vi "User Console.vi"(8 "error in (no error)":errorcluster, 10 "Queues":T3, 11 "UE Data Container":T4) -> (0 "error out":errorcluster)   [LabVIEW 2017]
doc: "The Process of ATM controller where user enters information and responds to system prompts.\n[Covers: UI1]"
uses:
  Shared Data/User Events/UE Data Container.ctl
  Error Handler/Controls/Error Data.ctl
  Controls/User Console - Transaction Enum.ctl
  Shared Data/Queues/Controls/Queues.ctl
  Controller/Controls/UI CMD.ctl
  Controller/Controls/Controller CMD.ctl
  Configuration/Controls/Config CMD.ctl
  Controls/User Console - Keypad.ctl
  Controls/User Console - Transactions.ctl
  Controls/User Console - References.ctl
panel:
  in  "Card Reader":bool
  in  "Transactions":T1
  in  "Keypad":T2
  # "[Covers: UI2]"
  # "[Covers: UI2B]"
  # "[Covers: UI2C]"
  # "[Covers: UI2A]"
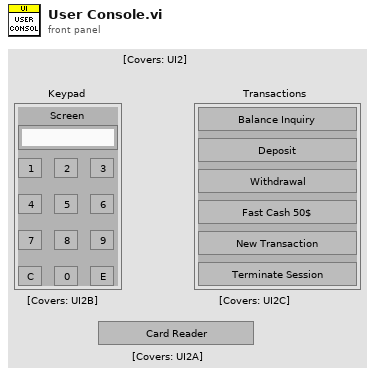
[diagram p1: front panel]
types:
  T1 = typedef "User Console - Transactions.ctl" = cluster{"Balance Inquiry":bool, "Deposit":bool, "Withdrawal":bool, "Fast Cash":bool, "New Transaction":bool, "Terminate":bool}
  T2 = typedef "User Console - Keypad.ctl" = cluster{"Screen":string, "1":bool, "2":bool, "3":bool, "4":bool, "5":bool, "6":bool, "7":bool, "8":bool, "9":bool, "C":bool, "0":bool, "E":bool}
  T3 = typedef "Queues.ctl" = cluster{"UI":refnum<queue>, "Controller":refnum<queue>, "Config":refnum<queue>, "User Console":refnum<queue>, "Display Console":refnum<queue>}
  T4 = typedef "UE Data Container.ctl" = cluster{"Stop UE":refnum<user-event>, "Stop DVR":refnum<data-value>, "Error UE":refnum<user-event>, "Deposit Change":refnum<user-event>, "Funds Change":refnum<user-event>, "Card Reader Change":refnum<user-event>, "Transaction Change":refnum<user-event>, "Keypad Screen Change":refnum<user-event>}
  T5 = typedef "User Console - References.ctl" = cluster{"Transactions":refnum<vi>, "Keypad":refnum<vi>, "Card Reader":refnum<vi>}
  T6 = typedef "User Console - Transaction Enum.ctl" = enum16{"Balance Inquiry", "Deposit", "Withdrawal", "Fat Cash", "New Transaction", "Terminate Session"}
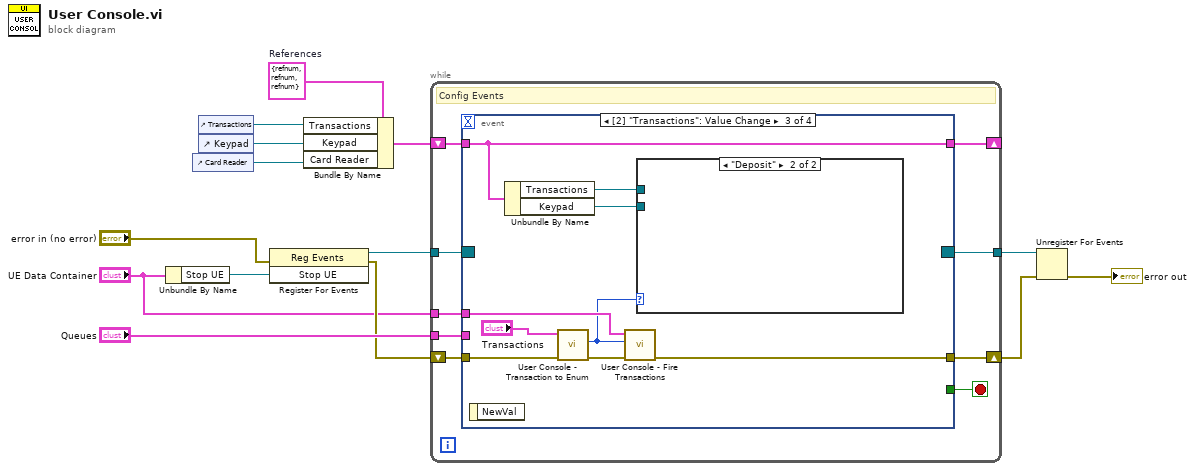
[diagram p0: block diagram]
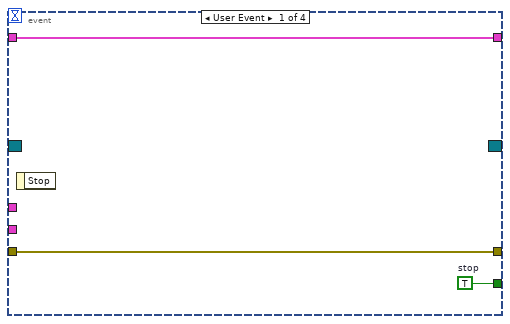
[diagram p2: hidden frame]
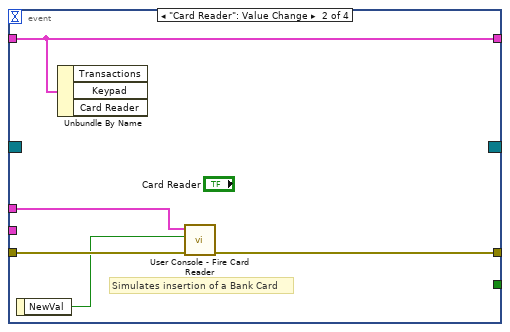
[diagram p3: hidden frame]
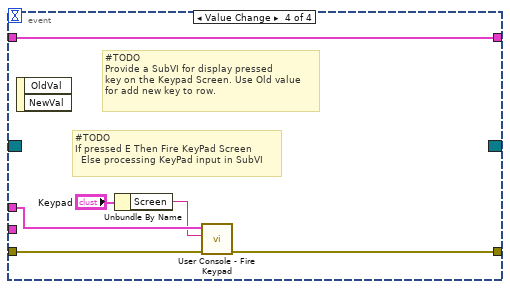
[diagram p5: hidden frame]
diagram:
  w6 = T5 {"Transactions"=refnum, "Keypad"=refnum, "Card Reader"=refnum}  # References
  n1 = Unbundle By Name("UE Data Container") -> ("Stop UE"=w14:refnum<user-event>)
  n2 = control-ref of="Card Reader"() -> (w3:refnum<vi>)
  n3 = control-ref of="Transactions"() -> (w5:refnum<vi>)
  n4 = control-ref of="Keypad"() -> (w4:refnum<vi>)
  n5 = register-events(error in="error in (no error)", w14) -> (reference out=w12:refnum<event-registration>, error out=w8:errorcluster)  [unwired: 1 in]
  n6 = Bundle By Name(cluster=w6, "Transactions"=w5, "Keypad"=w4, "Card Reader"=w3) -> (w2:T5)
  n7 = while {
    tunnel: w12 -> [w23]
    tunnel: [w22] -> w11
    tunnel: "Queues" -> [w20]
    shift-right: [w18] -> w10
    shift-left: w8 -> [w19]
    tunnel: "UE Data Container" -> [w17]
    shift-right: [w15] -> _
    shift-left: w2 -> [w16]
    stop <- w21 stop-if-true
    # "Config Events"
    n8 = event shown="[2] \"Transactions\": Value Change" {
      selector: w23 -> [_ _ _ _]
      dyn-events: [_ _ _ _] -> w22
      timeout: _ -> [_ _ _ _]
      tunnel: [w26 _ _ _] -> w21
      tunnel: w20 -> [_ _ _ _]
      tunnel: w19 -> [w24 w31 w40 w45]
      tunnel: [w24 w29 w37 w41] -> w18
      tunnel: w17 -> [_ w30 w39 w43]
      tunnel: w16 -> [w25 w27 w35 w46]
      tunnel: [w25 w27 w35 w46] -> w15
      event User Event {
        w26 = TRUE  # stop
        n9 = event-data() -> ()  [unwired: 1 in, 1 out]
      }
      event "Card Reader": Value Change {
        # "Simulates insertion of a Bank Card"
        n10 = event-data() -> ("NewVal"=w28:bool)  [unwired: 1 in]
        n11 = Unbundle By Name(w27) -> ()  [unwired: 3 out]
        n12 = call "User Console - Fire Card Reader.vi"("error in (no error)"=w31, "Card Reader Change"=w28, "UE Data Container"=w30) -> ("error out"=w29:errorcluster)  [unwired: 8 in]
      }
      event Value Change {
        n13 = event-data() -> ()  [unwired: 1 in, 1 out]
        n14 = Unbundle By Name(w35) -> ("Transactions"=w33:refnum<vi>, "Keypad"=w32:refnum<vi>)
        n15 = call "User Console - Transaction to Enum.vi"("error in (no error)"=w40, "Transactions"="Transactions") -> ("error out"=w38:errorcluster, "Transaction Enum"=w34:T6)  [unwired: 8 in]
        n16 = call "User Console - Fire Transactions.vi"("error in (no error)"=w38, "Transaction Enum"=w34, "UE Data Container"=w39) -> ("error out"=w37:errorcluster)  [unwired: 7 in, 1 out]
        n17 = case shown="\"Deposit\"" w34 {
          tunnel: w33 -> [_ _]
          tunnel: w32 -> [_ _]
          frame "Balance Inquiry", Default {
          }
          frame "Deposit" {
          }
        }
      }
      event Value Change {
        # "#TODO\nProvide a SubVI for display pressed\nkey on the Keypad Screen. Use Old value\nfor add new key to row."
        # "#TODO\nIf pressed E Then Fire KeyPad Screen\n  Else processing KeyPad input in SubVI"
        n18 = event-data() -> ()  [unwired: 1 in, 2 out]
        n19 = Unbundle By Name("Keypad") -> ("Screen"=w42:string)
        n20 = call "User Console - Fire Keypad.vi"("error in (no error)"=w45, "Keypad Screen"=w42, "UE Data Container"=w43) -> ("error out"=w41:errorcluster)  [unwired: 7 in, 1 out]
      }
    }
  }
  n21 = Unregister For Events(event registration refnum=w11, error in=w10) -> (error out=→"error out":errorcluster)
